vi "Read Cap Registers.vi"(11 "Toggle 6 in":refnum<class "Toggle 7.1.lvclass">) -> (2 "Cap Registers":T1[](array[typedef]), 3 "Toggle 6 out":refnum<class "Toggle 7.1.lvclass">)   [LabVIEW 2020, in "Toggle 7.1.lvclass"]
uses:
  Toggle 7.1.lvclass
  Controls/Capacitor register.ctl
  Toggle 7.1.lvclass/Toggle 7.1.ctl
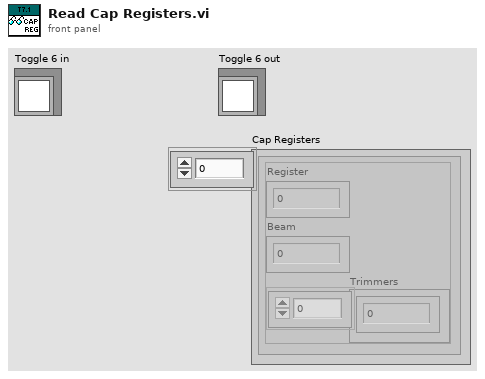
[diagram p1: front panel]
types:
  T1 = typedef "Toggle 7.1.lvclass/Capacitor register.ctl" = cluster{"Register":u32, "Beam":dbl, "Trimmers":dbl[]}
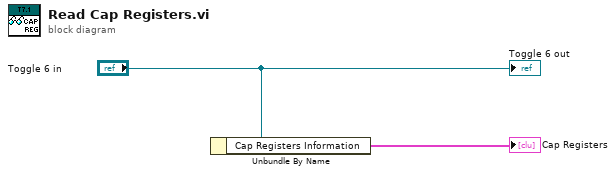
[diagram p0: block diagram]
diagram:
  n1 = Unbundle By Name("Toggle 6 in") -> ("Cap Registers Information"=→"Cap Registers":T1[])
  "Toggle 6 out" <- "Toggle 6 in"
